vi "CustomPID_v4.0.vi"(0 "PID Tuning Parameters":T1={"Kp"=0.1, "Ki"=0.1, "Kd"=0.1, "N-Diff"=10, "N-Int"=20, "Int Error Window"=0.5, "Max Ouput"=1.0, "Min Output"=-1.0} {"Int Error Window" min=0.0; "N-Int" min=2; "N-Diff" min=2; "Kd" min=0.0; "Ki" min=0.0; "Kp" min=0.0}, 1 "Goal":dbl(slide) scale=-1.0..1.0, 2 "Process Variable":dbl(slide) scale=-1.0..1.0, 3 "Custom Error Calculation":dbl(slide) scale=-1.0..1.0, 7 "Reset on Goal Change ?":bool, 9 "Use Custom Error Calculation ?":bool, 12 "Reinit":bool) -> (4 "Command":dbl format="%_4g", 6 "Is Reset":bool, 8 "Current Error":dbl format="%_4g", 15 "Controller Summary":T2(graph))   [LabVIEW 2019]
doc: "Brief PID Description:\n\nA good mechanical analogy for a PID algorithm is a spring-mass system with a viscous damper \n(https://ccrma.stanford.edu/CCRMA/Courses/150/img35.gif). The proportional term is the \"spring,\" it has the strongest influence when the robot system is furthest from its goal. The derivative term is the damping coefficient, it's what allows the system to stop oscillating and reach it's goal. The integral term mostly comes into play if the robot has been been trying to move for a lengthy amount of time but still isn't able to reach it's goal (this is referred to as steady-state error).\n\nRecommended Tuning Procedure:\n\n1) You may want to restrict the Max and Min Output parameters more than [-1, 1] during initial tuning to avoid damaging the system.\n2) If you do not wish to pre-calculate a Kp, carefully increase the Kp term from 0.0001 until the system starts moving.\n3) If the system is going the wrong direction, you may need to negate the Command.\n4) Continue inceasing Kp until the system oscillates about the Goal.\n5) Carefully increase Kd from 0.0001 until the system's response is sufficiently damped (i.e. until the oscillation is mitigated).\n6) Carefully increase Ki from 0.0001 to reduce the steady-state error (SSE) (if any).\n7) Adjust N-Diff if necessary (minimum of 2). Increasing N-Diff will reduce the effects of sensor (Process Variable) noise on the \nderivative term but will increase the lag on that component. You may also want to add a filter to Process Variable data.\n8) Adjust N-Int if necessary (minimum of 2). Increasing N-Int may help the system overcome SSE but may also increase integrator wind-up. It will also increase the lag for that component.\n9) Another way to reduce integrator wind-up is to set the Integral Error Window. The Intergral term will only be used if the magnitude of the error is less than the specified window.\n10) You may need to adjust Ki, and Kd after adjusting N-Diff and N-Int, respectively. \n\nAdditional Notes:\n\n1) Make sure that execution type for all instances of this VI are set to \"preallocated clone reentrant execution.\"\n2) Several parts of this VI were inspired by a PID algorithm written by Dr. Ira Hill at the University of Florida and have been developed in collaboration with FRC 2614.\n3) If you have any questions, feel free to contact me at lrscime.alpha@gmail.coms"
uses:
  <vilib>/Analysis/6fits.llb/Curve Fitting Criteria.ctl
  <vilib>/Analysis/NI_AALPro.lvlib
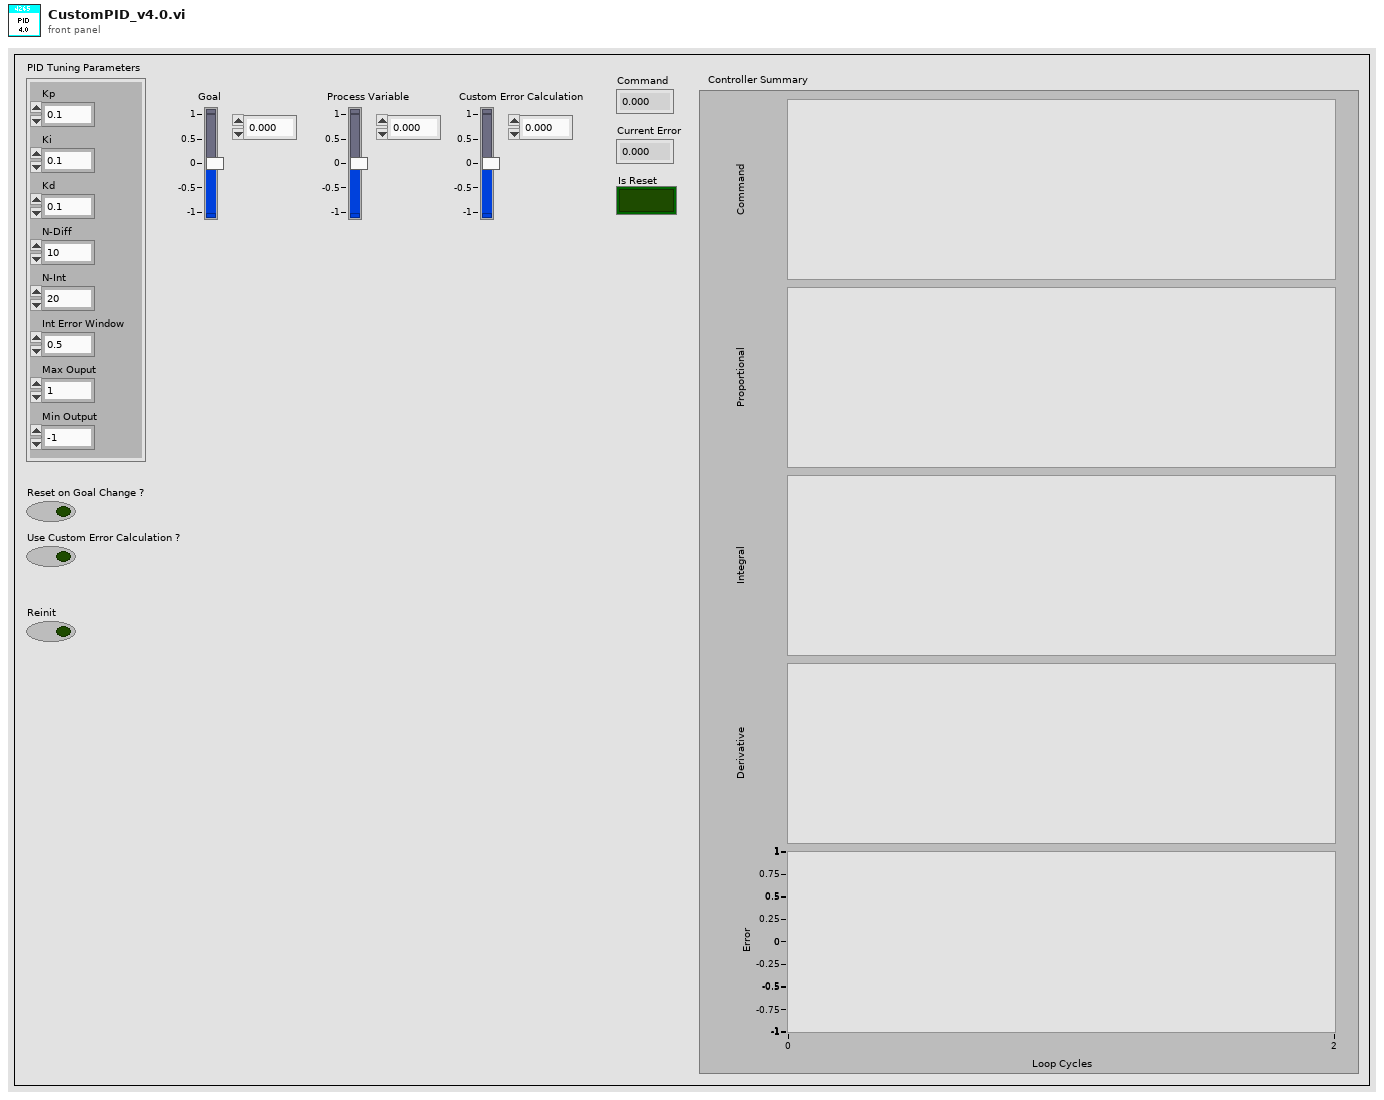
[diagram p1: front panel]
types:
  T1 = cluster{"Kp":dbl, "Ki":dbl, "Kd":dbl, "N-Diff":i32, "N-Int":i32, "Int Error Window":dbl, "Max Ouput":dbl, "Min Output":dbl}
  T2 = cluster{"Command":dbl, "Proportional":dbl, "Integral":dbl, "Derivative":dbl, "Goal":dbl}
  T3 = cluster{"Command":dbl, "Proportional":dbl, "Integral":dbl, "Derivative":dbl, "Error":dbl}
  T4 = typedef "NI_AALPro.lvlib/Curve Fitting Criteria.ctl" = u16
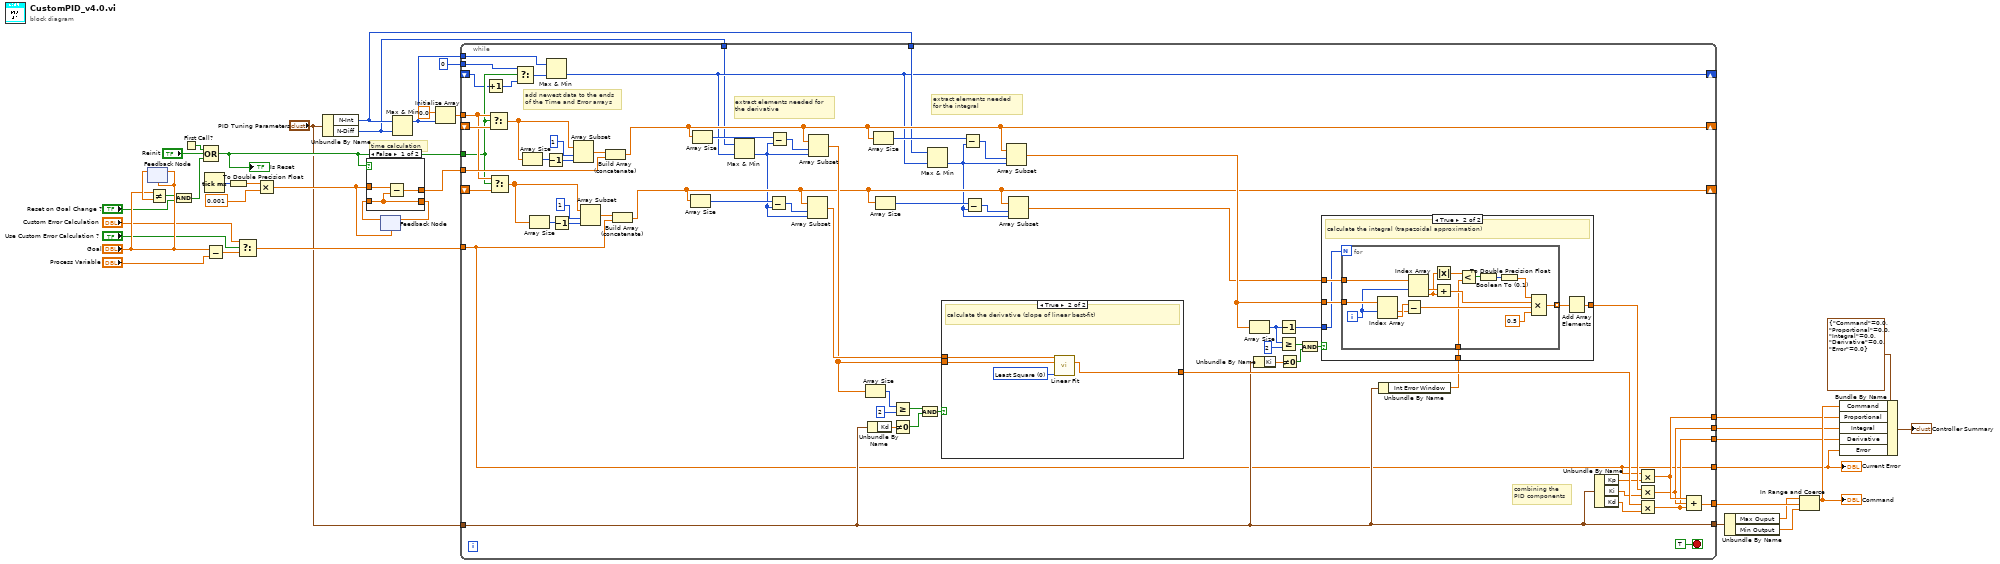
[diagram p0: block diagram]
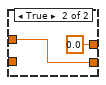
[diagram p2: hidden frame]
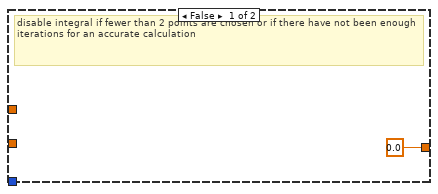
[diagram p3: hidden frame]
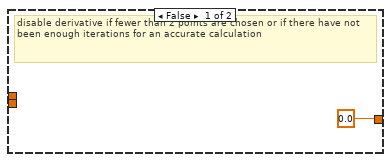
[diagram p4: hidden frame]
diagram:
  # "time calculation"
  n1 = feedback #1("Goal") -> (w33:dbl)
  n2 = feedback-in #1("Goal") -> ()
  n3 = Not Equal?(x="Goal", y=w33) -> (x != y?=w15:bool)
  n4 = And(x=w15, y="Reset on Goal Change ?") -> (x .and. y?=w26:bool)
  n5 = First Call?() -> (First Call?: T/F=w37:bool)
  n6 = Compound Arithmetic op=OR(w37, "Reinit", w26) -> (w27:bool)
  "Is Reset" <- w27
  n7 = Tick Count (ms)() -> (millisecond timer value=w32:u32)
  n8 = Subtract(x="Goal", y="Process Variable") -> (x-y=w13:dbl)
  n9 = To Double Precision Float(number=w32) -> (double precision float=w31:dbl)
  n10 = Select(t="Custom Error Calculation", s="Use Custom Error Calculation ?", f=w13) -> (s? t:f=w12:dbl)
  n11 = Multiply(x=w31, y=0.001) -> (x*y=w25:dbl)
  n12 = Unbundle By Name("PID Tuning Parameters") -> ("N-Int"=w6:i32, "N-Diff"=w5:i32)
  n13 = feedback #2(w25) -> (w28:dbl)
  n14 = case shown="False" w27 {
    tunnel: w25 -> [w41 w43]
    tunnel: [w39 w43] -> w29
    tunnel: [w40 0.0] -> w19
    tunnel: w28 -> [w39 _]
    frame False {
      n15 = Subtract(x=w41, y=w39) -> (x-y=w40:dbl)
    }
    frame True {
    }
  }
  n16 = feedback-in #2(w29) -> ()
  n17 = Max & Min(x=w6, y=w5) -> (max(x,y)=w7:i32)  [unwired: 1 out]
  n18 = Initialize Array(0.0 ("element"), w7) -> (w35:dbl[])
  n19 = while {
    tunnel: [w107] -> w38
    tunnel: w12 -> [w44]
    shift-right: [w88] -> _
    shift-left: _ -> [w81]
    tunnel: w19 -> [w102]
    shift-right: [w82] -> _
    shift-left: _ -> [w78]
    tunnel: w27 -> [w69]
    tunnel: w35 -> [w79]
    tunnel: [w44] -> w9
    tunnel: [w74] -> w23
    tunnel: [w73] -> w22
    tunnel: [w72] -> w21
    tunnel: 0 -> [w70]
    shift-right: [w53] -> _
    shift-left: _ -> [w67]
    tunnel: w7 -> [w64]
    tunnel: w6 -> [w54]
    tunnel: w5 -> [w52]
    tunnel: "PID Tuning Parameters" -> [w45]
    tunnel: [w45] -> w3
    stop <- TRUE stop-if-true
    # "combining the\nPID components"
    # "add newest data to the ends\nof the Time and Error arrays"
    # "extract elements needed for the integral"
    # "extract elements needed for the derivative"
    n20 = Increment(x=w67) -> (x+1=w68:i32)
    n21 = Select(t=w79, s=w69, f=w81) -> (s? t:f=w80:dbl[])
    n22 = Select(t=w79, s=w69, f=w78) -> (s? t:f=w77:dbl[])
    n23 = Select(t=w70, s=w69, f=w68) -> (s? t:f=w65:i32)
    n24 = Array Size(array=w80) -> (size(s)=w105:i32)
    n25 = Array Size(array=w77) -> (size(s)=w100:i32)
    n26 = Decrement(x=w105) -> (x-1=w104:i32)
    n27 = Max & Min(x=w64, y=w65) -> (min(x,y)=w53:i32)  [unwired: 1 out]
    n28 = Decrement(x=w100) -> (x-1=w99:i32)
    n29 = Array Subset(array=w80, index=1, length=w104) -> (w103:dbl[])
    n30 = Array Subset(array=w77, index=1, length=w99) -> (w98:dbl[])
    n31 = Build Array (concatenate)(w103, w102) -> (w88:dbl[])
    n32 = Build Array (concatenate)(w98, w44) -> (w82:dbl[])
    n33 = Array Size(array=w82) -> (size(s)=w94:i32)
    n34 = Array Size(array=w88) -> (size(s)=w97:i32)
    n35 = Max & Min(x=w52, y=w53) -> (min(x,y)=w66:i32)  [unwired: 1 out]
    n36 = Subtract(x=w94, y=w66) -> (x-y=w95:i32)
    n37 = Subtract(x=w97, y=w66) -> (x-y=w96:i32)
    n38 = Array Subset(array=w82, index=w95, length=w66) -> (w93:dbl[])
    n39 = Array Subset(array=w88, index=w96, length=w66) -> (w92:dbl[])
    n40 = Array Size(array=w92) -> (size(s)=w71:i32)
    n41 = Unbundle By Name(w45) -> ("Kd"=w51:dbl)
    n42 = Array Size(array=w88) -> (size(s)=w90:i32)
    n43 = Array Size(array=w82) -> (size(s)=w87:i32)
    n44 = Greater Or Equal?(x=w71, y=2) -> (x >= y?=w63:bool)
    n45 = Not Equal To 0?(x=w51) -> (x != 0?=w61:bool)
    n46 = Compound Arithmetic op=AND(w63, w61) -> (w62:bool)
    n47 = Max & Min(x=w54, y=w53) -> (min(x,y)=w60:i32)  [unwired: 1 out]
    n48 = case shown="True" w62 {
      tunnel: w93 -> [_ w136]
      tunnel: w92 -> [_ w135]
      tunnel: [0.0 w133] -> w75
      frame False {
        # "disable derivative if fewer than 2 points are chosen or if there have not been enough iterations for an accurate calculation"
      }
      frame True {
        w134 = T4 0 items=["Least Square", "Least Absolute Residual", "Bisquare"] ("method")
        # "calculate the derivative (slope of linear best-fit)"
        n49 = call <vilib>:"Linear Fit.vi"("Y"=w136, "X"=w135, "method"=w134) -> ("slope"=w133:dbl)  [unwired: 8 in, 4 out]
      }
    }
    n50 = Subtract(x=w90, y=w60) -> (x-y=w89:i32)
    n51 = Subtract(x=w87, y=w60) -> (x-y=w86:i32)
    n52 = Array Subset(array=w88, index=w89, length=w60) -> (w83:dbl[])
    n53 = Array Subset(array=w82, index=w86, length=w60) -> (w76:dbl[])
    n54 = Array Size(array=w83) -> (size(s)=w59:i32)
    n55 = Unbundle By Name(w45) -> ("Ki"=w50:dbl)
    n56 = Decrement(x=w59) -> (x-1=w58:i32)
    n57 = Greater Or Equal?(x=w59, y=2) -> (x >= y?=w57:bool)
    n58 = Not Equal To 0?(x=w50) -> (x != 0?=w55:bool)
    n59 = Compound Arithmetic op=AND(w57, w55) -> (w56:bool)
    n60 = Unbundle By Name(w45) -> ("Int Error Window"=w49:dbl)
    n61 = case shown="True" w56 {
      tunnel: [0.0 w110] -> w84
      tunnel: w83 -> [_ w115]
      tunnel: w76 -> [_ w114]
      tunnel: w49 -> [_ w113]
      tunnel: w58 -> [_ w112]
      frame False {
        # "disable integral if fewer than 2 points are chosen or if there have not been enough iterations for an accurate calculation"
      }
      frame True {
        # "calculate the integral (trapezoidal approximation)"
        n62 = for {
          N: w112 -> [_]
          tunnel: w115 -> [w131]
          tunnel: w114 -> [w125]
          tunnel: w113 -> [w118]
          tunnel: [w117] -> w111 mode=indexing
          i -> [w126]
          n63 = Index Array(array=w131, index #1=w126) -> (element #1=w129:dbl, element #2=w130:dbl)  [unwired: 1 in]
          n64 = Subtract(x=w130, y=w129) -> (x-y=w128:dbl)
          n65 = Index Array(array=w125, index #1=w126) -> (element #1=w123:dbl, element #2=w116:dbl)  [unwired: 1 in]
          n66 = Absolute Value(x=w116) -> (abs(x)=w122:dbl)
          n67 = Add(x=w123, y=w116) -> (x+y=w124:dbl)
          n68 = Less?(x=w122, y=w118) -> (x < y?=w121:bool)
          n69 = Boolean To (0,1)(Boolean=w121) -> (0, 1=w120:i16)
          n70 = To Double Precision Float(number=w120) -> (double precision float=w119:dbl)
          n71 = Compound Arithmetic op=MULTIPLY(w119, w124, w128, 0.5 ("value")) -> (w117:dbl)
        }
        n72 = Add Array Elements(numeric array=w111) -> (sum=w110:dbl)
      }
    }
    n73 = Unbundle By Name(w45) -> ("Kp"=w48:dbl, "Ki"=w47:dbl, "Kd"=w46:dbl)
    n74 = Multiply(x=w44, y=w48) -> (x*y=w74:dbl)
    n75 = Multiply(x=w84, y=w47) -> (x*y=w73:dbl)
    n76 = Multiply(x=w75, y=w46) -> (x*y=w72:dbl)
    n77 = Compound Arithmetic op=ADD(w74, w73, w72) -> (w107:dbl)
  }
  "Current Error" <- w9
  n78 = Unbundle By Name(w3) -> ("Max Ouput"=w2:dbl, "Min Output"=w1:dbl)
  n79 = In Range and Coerce(upper limit=w2, x=w38, lower limit=w1) -> (coerced(x)=w24:dbl)  [unwired: 1 out]
  "Command" <- w24
  n80 = Bundle By Name(cluster=T3 {"Command"=0.0, "Proportional"=0.0, "Integral"=0.0, "Derivative"=0.0, "Error"=0.0} ("input cluster"), "Command"=w24, "Proportional"=w23, "Integral"=w22, "Derivative"=w21, "Error"=w9) -> (→"Controller Summary":T3)
